vi "log_event_id.vi"(10 "Facility":string) -> (2 "Facility ID":i32)   [LabVIEW 2013]
uses:
  log_event.ctl
  initialization/micron_globals.vi
panel:
  # "Look up or allocate facilify ID for log_event call site.  Internal to log_event.vi.  This becomes index into \"Log Status\" global."
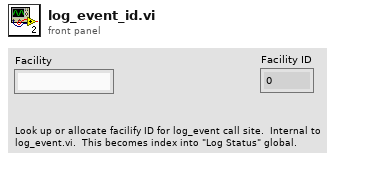
[diagram p1: front panel]
types:
  T1 = typedef "log_event.ctl" = cluster{"Facility ID":i32, "Severity":enum16{"OK", "Debug", "Warn", "Error"}, "Timestamp":timestamp, "Facility":string, "State":string, "Message":string}
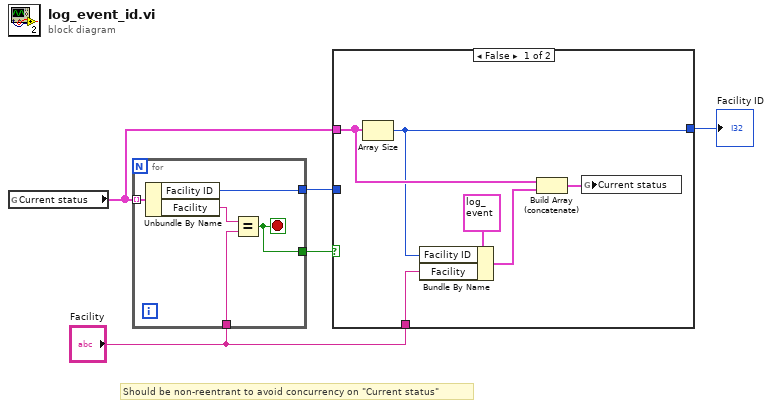
[diagram p0: block diagram]
diagram:
  # "Should be non-reentrant to avoid concurrency on \"Current status\""
  n1 = global read "micron_globals.vi" "Current status"() -> (w2:T1[])
  n2 = for {
    tunnel: w2 -> [w10] mode=indexing
    tunnel: [w8] -> w5
    tunnel: [w7] -> w4
    tunnel: "Facility" -> [w6]
    stop <- w8 stop-if-true
    n3 = Unbundle By Name(w10) -> ("Facility ID"=w7:i32, "Facility"=w9:string)
    n4 = Equal?(x=w9, y=w6) -> (x = y?=w8:bool)
  }
  n5 = case shown="False" w5 {
    tunnel: [w11 w17] -> w3
    tunnel: w4 -> [_ w17]
    tunnel: w2 -> [w14 _]
    tunnel: "Facility" -> [w15 _]
    frame False {
      n6 = Array Size(array=w14) -> (size(s)=w11:i32)
      n7 = Bundle By Name(cluster=T1 {"Facility ID"=0, "Severity"=enum."OK", "Timestamp"=timestamp(0 s since 1904-01-01), "Facility"="", "State"="", "Message"=""} ("input cluster"), "Facility ID"=w11, "Facility"=w15) -> (w13:T1)
      n8 = Build Array (concatenate)(w14, w13) -> (w12:T1[])
      n9 = global write "micron_globals.vi" "Current status"(w12) -> ()
    }
    frame True {
    }
  }
  "Facility ID" <- w3
